vi "Add ECAT Variable Contents.vi"(5 "Name Prefix":string, 7 "Add Name Property":bool, 8 "error in":errorcluster, 9 "Input Parent Ref in":T1 format="%.0x", 10 "Output Parent Ref in":T1 format="%.0x", 11 "IO Variable Container Contents":T2) -> (0 "error out":errorcluster)   [LabVIEW 2020, in "SEECD System Explorer.lvlib"]
uses:
  SEECD System Explorer.lvlib
  Type Defs/IOV Container Contents.ctl
  <vilib>/NI VeriStand/Custom Device API/Custom Device Item Ref.ctl
  <vilib>/NI VeriStand/Custom Device API/Custom Device Channel.ctl
  <vilib>/NI VeriStand/Custom Device API/Custom Device Channel Type.ctl
  Shared/Globals/Property Strings.vi
  Shared/Globals/Scan Engine GUIDs.vi
  <vilib>/NI VeriStand/Custom Device API/Set Item Property (String).vi
  <vilib>/NI VeriStand/Custom Device API/Custom Device API.lvlib
  Shared/SEECD Shared.lvlib
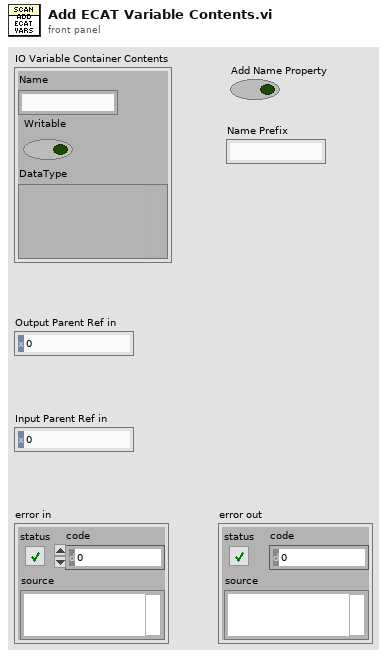
[diagram p1: front panel]
types:
  T1 = typedef "Custom Device API.lvlib/Custom Device Item Ref.ctl" = u64
  T2 = typedef "SEECD System Explorer.lvlib/IOV Container Contents.ctl" = cluster{"Name":string, "Writable":bool, "DataType":variant}
  T3 = typedef "Custom Device API.lvlib/Custom Device Channel.ctl" = cluster{"Type":T4, "Units":string, "Default Value":dbl, "Faultable":bool, "Scalable":bool}
  T4 = typedef "Custom Device API.lvlib/Custom Device Channel Type.ctl" = enum16{"Input", "Output"}
  T5 = typedef "SEECD Shared.lvlib/ECAT Channel Data Type.ctl" = enum16{"Boolean", "Fixed Point", "Int8", "Int16", "Int32", "Int64", "U32 Bit Field", "UInt8", "UInt16", "UInt32", "UInt64", "Other", "DBL", "SGL"}
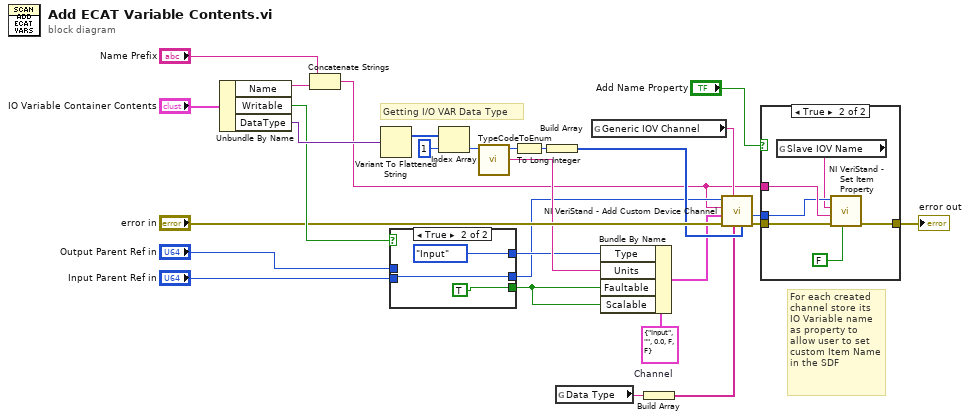
[diagram p0: block diagram]
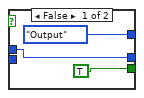
[diagram p3: hidden frame]
diagram:
  w4 = T3 {"Type"=enum."Input", "Units"="", "Default Value"=0.0, "Faultable"=FALSE, "Scalable"=FALSE}  # Channel
  # "For each created channel store its IO Variable name as property to allow user to set custom Item Name in the SDF"
  # "Getting I/O VAR Data Type"
  n1 = Unbundle By Name("IO Variable Container Contents") -> ("Name"=w26:string, "Writable"=w27:bool, "DataType"=w28:variant)
  n2 = Concatenate Strings("Name Prefix", w26) -> (w2:string)
  n3 = Variant To Flattened String(Variant=w28) -> (1:w7:i16[])  [unwired: 1 out]
  n4 = case shown="True" w27 {
    tunnel: [Custom_Device_Channel_Type."Output" ("Type") Custom_Device_Channel_Type."Input" ("Type")] -> w15
    tunnel: [w29 w32] -> w10
    tunnel: "Output Parent Ref in" -> [w29 _]
    tunnel: "Input Parent Ref in" -> [_ w32]
    tunnel: [TRUE TRUE] -> w12
    frame False {
    }
    frame True {
    }
  }
  n5 = Index Array(array=w7, index=1) -> (element=w17:i16)
  n6 = call "TypeCodeToEnum.vi"("Type Code (numbers in hexadecimal)"=w17) -> (2:"UDV Data Type"=w16:string, 3:"UDV Data Type"=w19:T5)  [unwired: 9 in]
  n7 = To Long Integer(number=w19) -> (32bit integer=w18:i32)
  n8 = Build Array(w18) -> (w14:i32[])
  n9 = global read "Property Strings.vi" "Data Type"() -> (w13:string)
  n10 = global read "Scan Engine GUIDs.vi" "Generic IOV Channel"() -> (w20:string)
  n11 = Bundle By Name(cluster=w4, "Type"=w15, "Units"=w16, "Faultable"=w12, "Scalable"=w12) -> (w5:T3)
  n12 = Build Array(w13) -> (w6:string[])
  n13 = call <vilib>:"NI VeriStand - Add Custom Device Channel.vi"("Property Values"=w14, "Property names"=w6, "GUID (Default Channel)"=w20, "error in (no error)"="error in", "Channel"=w5, "Channel Name"=w2, "Parent Ref in"=w10) -> ("error out"=w21:errorcluster, "Channel Ref"=w23:T1)  [unwired: 1 in, 2 out]
  n14 = case shown="True" "Add Name Property" {
    tunnel: w2 -> [_ w41]
    tunnel: w23 -> [_ w40]
    tunnel: [w35 w37] -> w22
    tunnel: w21 -> [w35 w36]
    frame False {
    }
    frame True {
      n15 = global read "Property Strings.vi" "Slave IOV Name"() -> (w39:string)
      n16 = call-poly <vilib>:"NI VeriStand - Set Item Property.vi"("Binary String (T)"=FALSE, "error in (no error)"=w36, "Value"=w41, "Property Name"=w39, "Item Ref in"=w40) -> ("error out"=w37:errorcluster)  [unwired: 4 in, 2 out]
    }
  }
  "error out" <- w22
